vi "Save Test Executive.vi"(6 "New GUIDs":bool, 7 "Root ID":string, 8 "error in (no error)":errorcluster, 9 "Indent":i32, 10 "Persistence in":refnum<class "IPersist.lvclass">, 11 "Test Executive in":refnum<class "Test Executive.lvclass">) -> (0 "error out":errorcluster, 1 "Flattened Test Executive":string[](array[string]), 2 "Persistence out":refnum<class "IPersist.lvclass">, 3 "Test Executive out":refnum<class "Test Executive.lvclass">)   [LabVIEW 2017, in "Test Executive.lvlib" / "Test Executive.lvclass"]
uses:
  <vilib>/gpm_packages/@cs/test-executive/Source/Test Executive/TestExecutive/Test Executive.lvclass
  <vilib>/gpm_packages/@cs/persistence/source/IPersist/IPersist.lvclass
  <vilib>/gpm_packages/@cs/test-executive/Source/Test Executive/TestExecutive/Test Executive.lvclass/Test Executive.ctl
  <vilib>/gpm_packages/@cs/test-executive/Source/Test Executive/Executioner/Executioner.lvclass
  <vilib>/gpm_packages/@cs/linked-list/Source/Linked List/Linked List Ref/Linked List Ref.lvclass
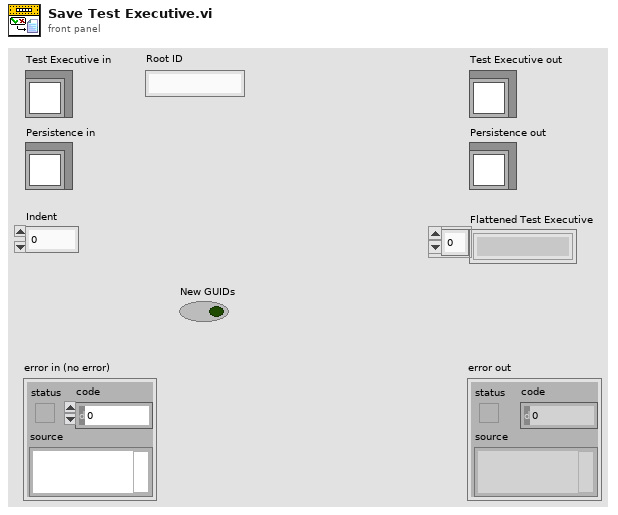
[diagram p1: front panel]
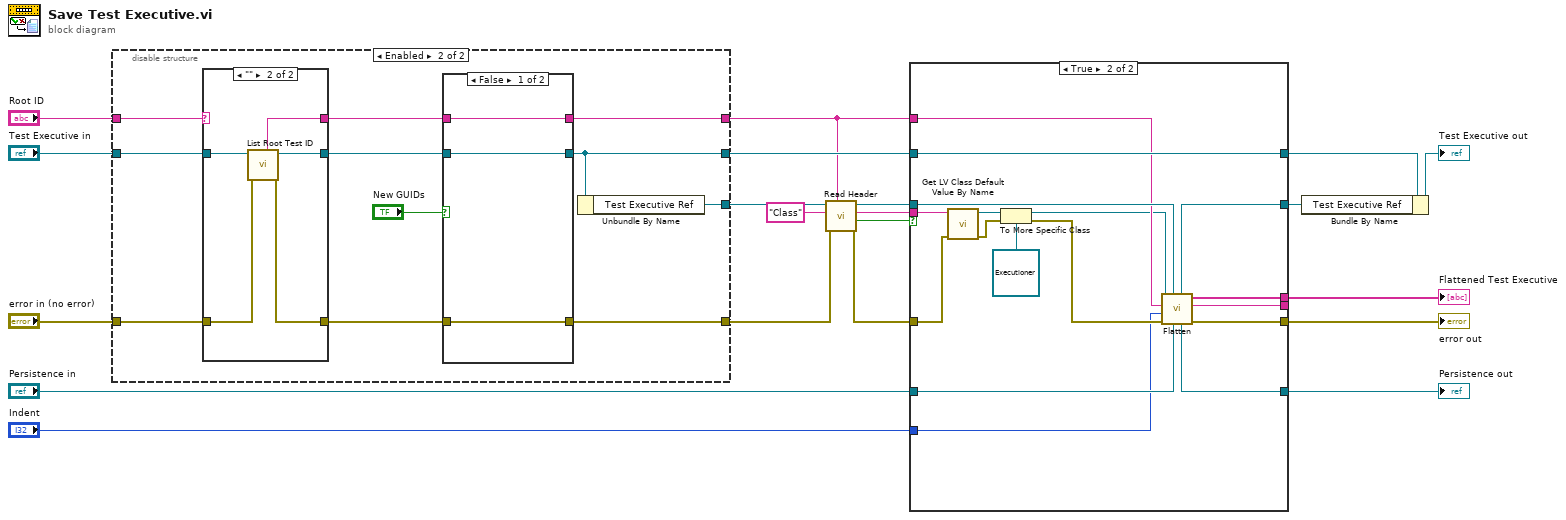
[diagram p0: block diagram]
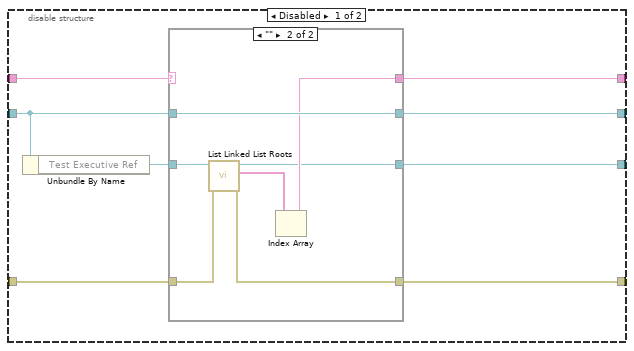
[diagram p2: hidden frame]
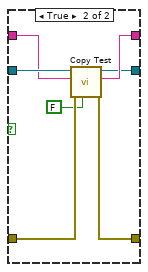
[diagram p4: hidden frame]
diagram:
  n1 = disable-structure shown="Enabled" {
    disable-tunnel: [w28 w41] -> w20
    disable-tunnel: [w27 w45] -> w16
    disable-tunnel: [w26 w42] -> w13
    disable-tunnel: [w25 w44] -> w12
    disable-tunnel: "error in (no error)" -> [w24 w50]
    disable-tunnel: "Test Executive in" -> [w23 w49]
    disable-tunnel: "Root ID" -> [w22 w48]
    frame Disabled {
      n2 = Unbundle By Name(w23) -> ("Test Executive Ref"=w21:refnum<data-value>)
      n3 = case shown="\"\"" w22 {
        selector: w22 -> [w31 _]
        tunnel: w23 -> [w32 w39]
        tunnel: w21 -> [w30 w38]
        tunnel: [w32 w39] -> w26
        tunnel: w24 -> [w29 w37]
        tunnel: [w31 w35] -> w25
        tunnel: [w30 w34] -> w28
        tunnel: [w29 w33] -> w27
        frame Default {
        }
        frame "" {
          n4 = call <vilib>:"List Linked List Roots.vi"("error in (no error)"=w37, "Linked List Ref"=w38) -> ("error out"=w33:errorcluster, "Root IDs"=w36:string[], "Linked List Ref out"=w34:refnum<data-value>)  [unwired: 6 in, 1 out]
          n5 = Index Array(array=w36) -> (element=w35:string)  [unwired: 1 in]
        }
      }
    }
    frame Enabled {
      n6 = case shown="\"\"" w48 {
        selector: w48 -> [w62 _]
        tunnel: w49 -> [w63 w68]
        tunnel: [w63 w67] -> w47
        tunnel: w50 -> [w61 w66]
        tunnel: [w62 w64] -> w43
        tunnel: [w61 w65] -> w46
        frame Default {
        }
        frame "" {
          n7 = call-dynamic "List Root Test ID.vi"("error in (no error)"=w66, "Test Executive in"=w68) -> ("error out"=w65:errorcluster, "Test Executive out"=w67:refnum<class "Test Executive.lvclass">, "Root ID"=w64:string)  [unwired: 5 in, 2 out]
        }
      }
      n8 = case shown="False" "New GUIDs" {
        tunnel: w47 -> [w53 w60]
        tunnel: w46 -> [w51 w59]
        tunnel: [w51 w58] -> w45
        tunnel: [w52 w56] -> w44
        tunnel: w43 -> [w52 w55]
        tunnel: [w53 w54] -> w42
        frame False {
        }
        frame True {
          n9 = call-dynamic "Copy Test.vi"("Move?"=FALSE, "error in (no error)"=w59, "Test ID"=w55, "Test Executive in"=w60) -> ("error out"=w58:errorcluster, "Test ID out"=w56:string, "Test Executive out"=w54:refnum<class "Test Executive.lvclass">)  [unwired: 5 in]
        }
      }
      n10 = Unbundle By Name(w42) -> ("Test Executive Ref"=w41:refnum<data-value>)
    }
  }
  n11 = call <vilib>:"Read Header.vi"("Linked List ID"=w12, "error in (no error)"=w16, "Header Name"="Class", "Linked List Ref"=w20) -> ("error out"=w17:errorcluster, "found"=w18:bool, "Header Value"=w14:string, "Linked List Ref out"=w15:refnum<data-value>)  [unwired: 4 in]
  n12 = case shown="True" w18 {
    tunnel: w17 -> [w71 w86]
    tunnel: w15 -> [w72 w77]
    tunnel: w14 -> [_ w89]
    tunnel: w13 -> [w73 w90]
    tunnel: [w73 w90] -> w5
    tunnel: [w72 w83] -> w7
    tunnel: [w71 w84] -> w10
    tunnel: w12 -> [w70 w76]
    tunnel: [w70 w82] -> _
    tunnel: [_ w81] -> w2
    tunnel: "Persistence in" -> [w69 w78]
    tunnel: [w69 w80] -> w3
    tunnel: "Indent" -> [_ w74]
    frame False {
    }
    frame True {
      n13 = call <vilib>:"Get LV Class Default Value By Name.vi"("error in (no error)"=w86, "class name"=w89) -> ("error out"=w85:errorcluster, "object"=w88:refnum<class>)  [unwired: 8 in]
      n14 = To More Specific Class(target class=refnum<class "Executioner.lvclass"> refnum ("Test Executive.lvlib:Executioner.lvclass"), reference=w88, error in=w85) -> (specific class reference=w75:refnum<class "Executioner.lvclass">, error out=w79:errorcluster)
      n15 = call-dynamic "Flatten.vi"("Persistence in"=w78, "Linked List Ref"=w77, "error in (no error)"=w79, "Indent"=w74, "Active Unique ID"=w76, "Executioner in"=w75) -> ("error out"=w84:errorcluster, "Active Unique ID out"=w82:string, "Flattened Test Executive"=w81:string[], "Persistence out"=w80:refnum<class "IPersist.lvclass">, "Linked List Ref out"=w83:refnum<data-value>)  [unwired: 1 in]
    }
  }
  "error out" <- w10
  "Persistence out" <- w3
  "Flattened Test Executive" <- w2
  n16 = Bundle By Name(cluster=w5, "Test Executive Ref"=w7) -> (→"Test Executive out":refnum<class "Test Executive.lvclass">)
